vi "Subtract Polynomials (CDB).vi"(8 "threshold type":T1 items=["Absolute Value", "Relative Value"], 9 "threshold":dbl, 10 "Q(x)":cdb[](array[numeric]) format="%#.6g", 11 "P(x)":cdb[](array[numeric]) format="%#.6g") -> (0 "error":i32, 3 "P(x)-Q(x)":cdb[](array[numeric]) format="%#.6g")   [LabVIEW 2017, in "NI_AALPro.lvlib"]
doc: "Subtracts polynomial <B>Q(x)</B> from polynomial <B>P(x)</B>. The data types you wire to the <B>P(x)</B> and <B>Q(x)</B> inputs determine the polymorphic instance to use."
uses:
  NI_AALPro.lvlib
  Remove Zero Threshold Type.ctl
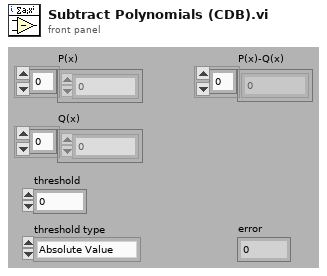
[diagram p1: front panel]
types:
  T1 = typedef "NI_AALPro.lvlib/Remove Zero Threshold Type.ctl" = u16
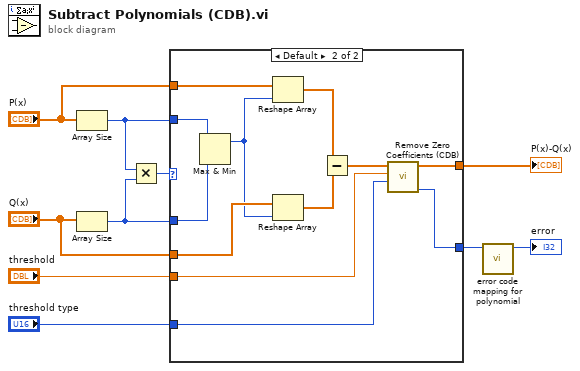
[diagram p0: block diagram]
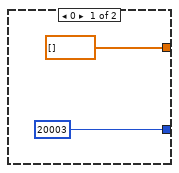
[diagram p2: hidden frame]
diagram:
  n1 = Array Size(array="P(x)") -> (size(s)=w7:i32)
  n2 = Array Size(array="Q(x)") -> (size(s)=w6:i32)
  n3 = Multiply(x=w7, y=w6) -> (x*y=w5:i32)
  n4 = case shown="Default" w5 {
    tunnel: w7 -> [_ w24]
    tunnel: w6 -> [_ w23]
    tunnel: "P(x)" -> [_ w16]
    tunnel: "Q(x)" -> [_ w19]
    tunnel: [cdb[] [] w21] -> w8
    tunnel: [20003 ("empty array") w20] -> w4
    tunnel: "threshold" -> [_ w14]
    tunnel: "threshold type" -> [_ w13]
    frame 0 {
    }
    frame Default {
      n5 = Max & Min(x=w24, y=w23) -> (max(x,y)=w17:i32)  [unwired: 1 out]
      n6 = Reshape Array(w16, w17) -> (w15:cdb[])
      n7 = Reshape Array(w19, w17) -> (w18:cdb[])
      n8 = Subtract(x=w15, y=w18) -> (x-y=w22:cdb[])
      n9 = call "Remove Zero Coefficients (CDB).vi"("threshold type"=w13, "threshold"=w14, "P(x) In"=w22) -> ("error"=w20:i32, "P(x) Out"=w21:cdb[])  [unwired: 6 in, 1 out]
    }
  }
  "P(x)-Q(x)" <- w8
  n10 = call "error code mapping for polynomial.vi"("error in"=w4) -> ("error out"=→"error":i32)  [unwired: 10 in]
